vi "svc_Get Strings that Match Substring Expression.vi"(8 "substring 2":string, 9 "separator":string, 10 "substring1":string, 11 "strings":string[](array[string])) -> (3 "matching strings":string[](array[string]))   [LabVIEW 2017]
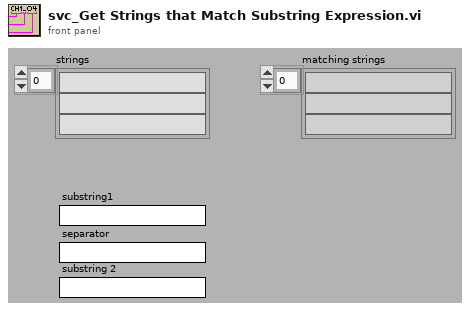
[diagram p1: front panel]
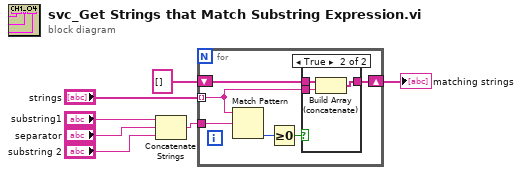
[diagram p0: block diagram]
diagram:
  n1 = Concatenate Strings("substring1", "separator", "substring 2") -> (w5:string)
  n2 = for {
    tunnel: "strings" -> [w8] mode=indexing
    tunnel: w5 -> [w13]
    shift-right: [w10] -> w7
    shift-left: string[] [] -> [w9]
    n3 = Match Pattern(string=w8, regular expression=w13) -> (offset past match=w12:i32)  [unwired: 1 in, 3 out]
    n4 = Greater Or Equal To 0?(x=w12) -> (x >= 0?=w11:bool)
    n5 = case shown="True" w11 {
      tunnel: w8 -> [_ w17]
      tunnel: [w14 w16] -> w10
      tunnel: w9 -> [w14 w15]
      frame False {
      }
      frame True {
        n6 = Build Array (concatenate)(w15, w17) -> (w16:string[])
      }
    }
  }
  "matching strings" <- w7
